vi "Retrieve Full Scale.vi"(8 "error in":errorcluster, 10 "Model Data":string, 11 "Alicat Device in":refnum<class "Alicat Device.lvclass">) -> (0 "error out":errorcluster, 1 "Type":string, 2 "Full Scale":sgl, 3 "Alicat Device out":refnum<class "Alicat Device.lvclass">)   [LabVIEW 2019, in "Alicat Device.lvclass"]
doc: "The full scale of the device defines the input command for the setpoint (if the device is a controller). The setpoint command will use the full scale (FS) such that \n\nVal = SP*64000/FS"
uses:
  Alicat Device.lvclass
  Alicat Device.lvclass/Alicat Device.ctl
  <vilib>/NI/Tools/String/Tools_String.lvlib
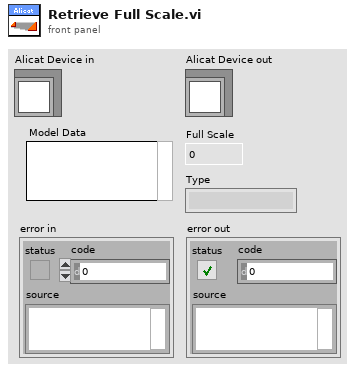
[diagram p1: front panel]
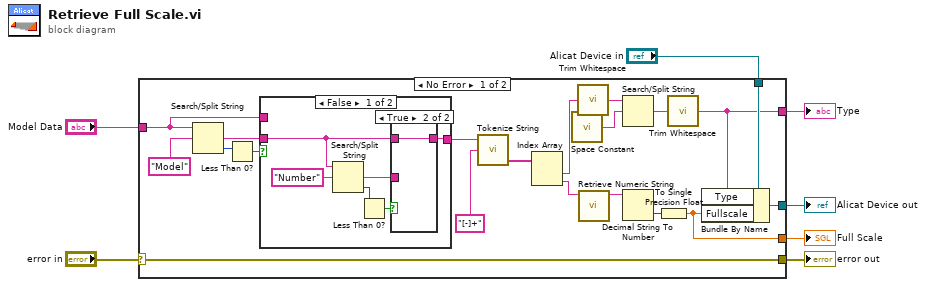
[diagram p0: block diagram]
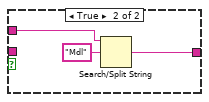
[diagram p3: hidden frame]
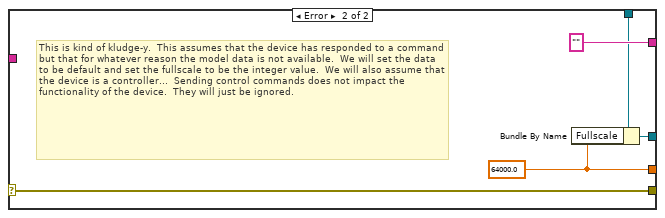
[diagram p4: hidden frame]
diagram:
  n1 = case shown="No Error" "error in" {
    selector: "error in" -> [w8 w39]
    tunnel: "Model Data" -> [w18 _]
    tunnel: "Alicat Device in" -> [w12 w42]
    tunnel: [w11 w41] -> w5
    tunnel: [w10 "" ("trimmed string")] -> w4
    tunnel: [w9 w40] -> w2
    tunnel: [w8 w39] -> w1
    frame No Error {
      n2 = Search/Split String(string=w18, search string/char (-)="Model") -> (match + rest of string=w24:string, offset of match=w26:i32)  [unwired: 1 in, 1 out]
      n3 = Less Than 0?(x=w26) -> (x < 0?=w25:bool)
      n4 = case shown="False" w25 {
        tunnel: w18 -> [_ w38]
        tunnel: w24 -> [w30 _]
        tunnel: [w29 w36] -> w23
        frame False {
          n5 = Search/Split String(string=w30, search string/char (-)="Number") -> (match + rest of string=w28:string, offset of match=w32:i32)  [unwired: 1 in, 1 out]
          n6 = Less Than 0?(x=w32) -> (x < 0?=w31:bool)
          n7 = case shown="True" w31 {
            tunnel: w30 -> [_ w35]
            tunnel: [w34 w35] -> w29
            tunnel: w28 -> [w34 _]
            frame False {
            }
            frame True {
            }
          }
        }
        frame True {
          n8 = Search/Split String(string=w38, search string/char (-)="Mdl") -> (match + rest of string=w36:string)  [unwired: 1 in, 2 out]
        }
      }
      n9 = call <vilib>:"Tokenize String.vi"("delimiter ([\\s\\t\\n\\r]+)"="[-]+" ("delimiter ([\\s\\t\\n\\r]+)"), "input string"=w23) -> ("token array"=w21:string[])  [unwired: 2 in, 1 out]
      n10 = Index Array(array=w21) -> (element #1=w16:string, element #2=w17:string)  [unwired: 2 in]
      n11 = call <vilib>:"Space Constant.vi"() -> ("String"=w14:string)
      n12 = call <vilib>:"Trim Whitespace.vi"("string"=w16) -> ("trimmed string"=w15:string)  [unwired: 1 in]
      n13 = call "Retrieve Numeric String.vi"("String in"=w17) -> ("Numeric String"=w20:string)  [unwired: 10 in]
      n14 = Search/Split String(string=w15, search string/char (-)=w14) -> (match + rest of string=w13:string)  [unwired: 1 in, 2 out]
      n15 = Decimal String To Number(string=w20) -> (number=w19:i32)  [unwired: 2 in, 1 out]
      n16 = To Single Precision Float(number=w19) -> (single precision float=w9:sgl)
      n17 = call <vilib>:"Trim Whitespace.vi"("string"=w13) -> ("trimmed string"=w10:string)  [unwired: 1 in]
      n18 = Bundle By Name(cluster=w12, "Type"=w10, "Fullscale"=w9) -> (w11:refnum<class "Alicat Device.lvclass">)
    }
    frame Error {
      w40 = sgl 64000.0
      # "This is kind of kludge-y.  This assumes that the device has responded to a command but that for whatever reason the model data is not available.  We will set the data to be default and set the fullscale to be the integer value.  We will also assume that the device is a controller...  Sending control commands does not impact the functionality of the device.  They will just be ignored."
      n19 = Bundle By Name(cluster=w42, "Fullscale"=w40) -> (w41:refnum<class "Alicat Device.lvclass">)
    }
  }
  "Type" <- w4
  "Alicat Device out" <- w5
  "error out" <- w1
  "Full Scale" <- w2
